vi "rszvl_core_global.vi"() -> ()   [LabVIEW 2014] (continued)
"*WAI"=FALSE}, "Check Status Callback"=""}, {"Level"=3, "Descriptive Name"="NWA Distance To Fault Auto Number Of Points", "Class Only"=FALSE, "Data Type"=4, "Access"=1, "Identifier"="RSZVL_ATTR_NWA_DFAULT_POINTS", "Range Table"="", "Command"="CALC{Channel}:TRAN:DTF:POIN", "Read Callback"="", "Write Callback"="", "Range Callback"="", "Check Callback"="", "Rngtable Callback"="", "Coerce Callback"="", "User Callback"="", "Supported Models"="", "Instrument Options"="", "Repeated Capabilities"="", "Restricted Repeated Capabilities"="", "Help"="This attribute starts the automatic calculation of the number of points.\n\nAvailable Repeated Capabilities:\nChannel: CH1,CH2,CH3,CH4,CH5,CH6,CH7,CH8,CH9,CH10,CH11,CH12,CH13,CH14,CH15,CH16,CH17,CH18,CH19,CH20\r\n\nRemote-control command(s):\nCALCulate<Chn>:TRANsform:DTFault:POINts", "Flags"={"OPC Wait"=FALSE, "Dont check status"=FALSE, "*WAI"=FALSE}, "Check Status Callback"=""}, {"Level"=3, "Descriptive Name"="NWA Distance To Fault Select Cable", "Class Only"=FALSE, "Data Type"=2, "Access"=2, "Identifier"="RSZVL_ATTR_NWA_DFAULT_SELECT_CABLE", "Range Table"="", "Command"="CALC{Channel}:TRAN:DTF:SEL", "Read Callback"="", "Write Callback"="rszvl_quotedString_WriteCallback.vi", "Range Callback"="", "Check Callback"="", "Rngtable Callback"="", "Coerce Callback"="", "User Callback"="", "Supported Models"="", "Instrument Options"="", "Repeated Capabilities"="", "Restricted Repeated Capabilities"="", "Help"="This attribute selects a standard cable or a previously defined cable identified by its name.\n\nAvailable Repeated Capabilities:\nChannel: CH1,CH2,CH3,CH4,CH5,CH6,CH7,CH8,CH9,CH10,CH11,CH12,CH13,CH14,CH15,CH16,CH17,CH18,CH19,CH20\r\n\nRemote-control command(s):\nCALCulate<Chn>:TRANsform:DTFault:SELect '<cable name>'", "Flags"={"OPC Wait"=FALSE, "Dont check status"=FALSE, "*WAI"=FALSE}, "Check Status Callback"=""}, {"Level"=3, "Descriptive Name"="NWA Distance To Fault Delete Cable", "Class Only"=FALSE, "Data Type"=2, "Access"=1, "Identifier"="RSZVL_ATTR_NWA_DFAULT_DELETE_CABLE", "Range Table"="", "Command"="CALC{Channel}:TRAN:DTF:DEL", "Read Callback"="rszvl_quotedString_ReadCallback.vi", "Write Callback"="rszvl_quotedString_WriteCallback.vi", "Range Callback"="", "Check Callback"="", "Rngtable Callback"="", "Coerce Callback"="", "User Callback"="", "Supported Models"="", "Instrument Options"="", "Repeated Capabilities"="", "Restricted Repeated Capabilities"="", "Help"="This attribute deletes a previously defined cable identified by its name.\n\nAvailable Repeated Capabilities:\nChannel: CH1,CH2,CH3,CH4,CH5,CH6,CH7,CH8,CH9,CH10,CH11,CH12,CH13,CH14,CH15,CH16,CH17,CH18,CH19,CH20\r\n\nRemote-control command(s):\nCALCulate<Chn>:TRANsform:DTFault:DELete '<cable name>'", "Flags"={"OPC Wait"=FALSE, "Dont check status"=FALSE, "*WAI"=FALSE}, "Check Status Callback"=""}, {"Level"=3, "Descriptive Name"="NWA Distance To Fault Save Cable", "Class Only"=FALSE, "Data Type"=2, "Access"=1, "Identifier"="RSZVL_ATTR_NWA_DFAULT_SAVE_CABLE", "Range Table"="", "Command"="MMEM:STOR:CABL", "Read Callback"="", "Write Callback"="rszvl_quotedString_WriteCallback.vi", "Range Callback"="", "Check Callback"="", "Rngtable Callback"="", "Coerce Callback"="", "User Callback"="", "Supported Models"="", "Instrument Options"="", "Repeated Capabilities"="", "Restricted Repeated Capabilities"="", "Help"="This attribute copies all pre-defined and user-defined cable description files (*.rsc) to a specified directory. The contents of the source directories for cable description files (C:\\R_S\\Instr\\resources\\Nwa\\CableTypes for predefined, C:\\R_S\\Instr\\user\\Nwa\\CableTypes for user-defined cables) are not affected.\n\nAvailable Repeated Capabilities:\nNone\n\nRemote-control command(s):\nMMEMory:STORe:CABLe '<target_directory>'", "Flags"={"OPC Wait"=FALSE, "Dont check status"=FALSE, "*WAI"=FALSE}, "Check Status Callback"=""}, {"Level"=3, "Descriptive Name"="NWA Distance To Fault Load Cable", "Class Only"=FALSE, "Data Type"=2, "Access"=1, "Identifier"="RSZVL_ATTR_NWA_DFAULT_LOAD_CABLE", "Range Table"="", "Command"="MMEM:LOAD:CABL", "Read Callback"="", "Write Callback"="rszvl_quotedString_WriteCallback.vi", "Range Callback"="", "Check Callback"="", "Rngtable Callback"="", "Coerce Callback"="", "User Callback"="", "Supported Models"="", "Instrument Options"="", "Repeated Capabilities"="", "Restricted Repeated Capabilities"="", "Help"="This attribute loads all cable description files (*.rsc) from a specified directory. The default source directories for cable\ndescription files (C:\\R_S\\Instr\\resources\\Nwa\\CableTypes for predefined, C:\\R_S\\Instr\\user\\Nwa\\CableTypes for user-defined cables) are not affected.\n\nAvailable Repeated Capabilities:\nNone\n\nRemote-control command(s):\nMMEMory:LOAD:CABLe '<source_directory>'", "Flags"={"OPC Wait"=FALSE, "Dont check status"=FALSE, "*WAI"=FALSE}, "Check Status Callback"=""}, {"Level"=3, "Descriptive Name"="Fault Limit Check", "Class Only"=TRUE, "Data Type"=0, "Access"=0, "Identifier"="", "Range Table"="", "Command"="", "Read Callback"="", "Write Callback"="", "Range Callback"="", "Check Callback"="", "Rngtable Callback"="", "Coerce Callback"="", "User Callback"="", "Supported Models"="", "Instrument Options"="", "Repeated Capabilities"="", "Restricted Repeated Capabilities"="", "Help"="Put a help here", "Flags"={"OPC Wait"=FALSE, "Dont check status"=FALSE, "*WAI"=FALSE}, "Check Status Callback"=""}, {"Level"=4, "Descriptive Name"="NWA Fault Limit Check", "Class Only"=FALSE, "Data Type"=3, "Access"=2, "Identifier"="RSZVL_ATTR_NWA_FAULT_LIMIT_CHECK", "Range Table"="", "Command"="CALC{Channel}:TRAN:DTF:PEAK:STAT", "Read Callback"="", "Write Callback"="", "Range Callback"="", "Check Callback"="", "Rngtable Callback"="", "Coerce Callback"="", "User Callback"="", "Supported Models"="", "Instrument Options"="", "Repeated Capabilities"="", "Restricted Repeated Capabilities"="", "Help"="This attribute enables or disables the fault limit check.\n\nAvailable Repeated Capabilities:\nChannel: CH1,CH2,CH3,CH4,CH5,CH6,CH7,CH8,CH9,CH10,CH11,CH12,CH13,CH14,CH15,CH16,CH17,CH18,CH19,CH20\r\n\nRemote-control command(s):\nCALCulate<Chn>:TRANsform:DTFault:PEAK:STATe ON | OFF", "Flags"={"OPC Wait"=FALSE, "Dont check status"=FALSE, "*WAI"=FALSE}, "Check Status Callback"=""}, {"Level"=4, "Descriptive Name"="NWA Fault Threshold", "Class Only"=FALSE, "Data Type"=1, "Access"=2, "Identifier"="RSZVL_ATTR_NWA_FAULT_THRESHOLD", "Range Table"="", "Command"="CALC{Channel}:TRAN:DTF:PEAK:THR", "Read Callback"="", "Write Callback"="", "Range Callback"="", "Check Callback"="", "Rngtable Callback"="", "Coerce Callback"="", "User Callback"="", "Supported Models"="", "Instrument Options"="", "Repeated Capabilities"="", "Restricted Repeated Capabilities"="", "Help"="This attribute specify a fault limit.\n\nAvailable Repeated Capabilities:\nChannel: CH1,CH2,CH3,CH4,CH5,CH6,CH7,CH8,CH9,CH10,CH11,CH12,CH13,CH14,CH15,CH16,CH17,CH18,CH19,CH20\r\n\nRemote-control command(s):\nCALCulate<Chn>:TRANsform:DTFault:PEAK:THReshold", "Flags"={"OPC Wait"=FALSE, "Dont check status"=FALSE, "*WAI"=FALSE}, "Check Status Callback"=""}, {"Level"=4, "Descriptive Name"="NWA Fault Peak Count", "Class Only"=FALSE, "Data Type"=0, "Access"=0, "Identifier"="RSZVL_ATTR_NWA_FAULT_PEAK_COUNT", "Range Table"="", "Command"="CALC{Channel}:TRAN:DTF:PEAK:COUN?", "Read Callback"="", "Write Callback"="", "Range Callback"="", "Check Callback"="", "Rngtable Callback"="", "Coerce Callback"="", "User Callback"="", "Supported Models"="", "Instrument Options"="", "Repeated Capabilities"="", "Restricted Repeated Capabilities"="", "Help"="This attribute returns the number of peaks on the active distance trace which are above the fault limit (CALCulate<Chn>:TRANsform:DTFault:PEAK:THReshold).\n\nAvailable Repeated Capabilities:\nChannel: CH1,CH2,CH3,CH4,CH5,CH6,CH7,CH8,CH9,CH10,CH11,CH12,CH13,CH14,CH15,CH16,CH17,CH18,CH19,CH20\r\n\nRemote-control command(s):\nCALCulate<Chn>:TRANsform:DTFault:PEAK:COUNt?", "Flags"={"OPC Wait"=FALSE, "Dont check status"=FALSE, "*WAI"=FALSE}, "Check Status Callback"=""}, {"Level"=1, "Descriptive Name"="NWA Display Control", "Class Only"=TRUE, "Data Type"=0, "Access"=0, "Identifier"="", "Range Table"="", "Command"="", "Read Callback"="", "Write Callback"="", "Range Callback"="", "Check Callback"="", "Rngtable Callback"="", "Coerce Callback"="", "User Callback"="", "Supported Models"="", "Instrument Options"="", "Repeated Capabilities"="", "Restricted Repeated Capabilities"="", "Help"="(1) NWA Color Scheme:\nThis attribute selects the color scheme for all diagram areas in the active setup.\n\n(2) NWA Frequency Info State:\nThis attribute activates/deactivates the display of the frequency information. For example to protect confidential data it can be useful to hide the frequency information.\n\n(3) NWA Trace Color State:\nThis attribute defines the trace color schemes in different diagram areas.\n\n(4) NWA Marker Color State:\nThis attribute displays all markers with the same color or display each marker with the color of the associated trace.\n\n(5) NWA Save Color Scheme:\nThis attribute stores a color scheme to a specified NWA color scheme file.\n\n(6) NWA Load Color Scheme:\nThis attribute loads a color scheme from a specified NWA color scheme file.\n\n(7) NWA Display Update:\nThis attribute switches the display on or off while the analyzer is in the remote state. The attribute has no effect while the analyzer is in the Local operating state.\n\n(8) NWA Error Display State:\nThis attribute switches the display of a tooltip for remote command errors on or off. The tooltip appears at the bottom of the remote screen and of the manual screen.\n\n(9) NWA Remote Display Title:\nThis attribute defines a title for the remote display.\n\n(10) NWA Diagram Area State:\nThis attribute creates or deletes a diagram area, identified by its area number <Wnd>.\n\n(11) NWA Diagram Area Maximize:\nThis attribute maximizes all diagram areas in the active setup or restores the previous display configuration. It acts on all diagrams of the current setup, however, the diagram no. <Wnd> is displayed on top of the others.\n\n(12) NWA Diagram Area Title State:\nThis attribute displays or hides the title for area number <Wnd>, defined by means of DISPlay:WINDow<Wnd>:TITLe:DATA.\n\n(13) NWA Diagram Area Title:\nThis attribute defines a title for diagram area <Wnd>.", "Flags"={"OPC Wait"=FALSE, "Dont check status"=FALSE, "*WAI"=FALSE}, "Check Status Callback"=""}, {"Level"=2, "Descriptive Name"="NWA Color Scheme", "Class Only"=FALSE, "Data Type"=0, "Access"=2, "Identifier"="RSZVL_ATTR_NWA_COLOR_SCHEME", "Range Table"="rszvl_rngNWAColorScheme", "Command"="SYST:DISP:COL", "Read Callback"="", "Write Callback"="", "Range Callback"="", "Check Callback"="", "Rngtable Callback"="", "Coerce Callback"="", "User Callback"="", "Supported Models"="", "Instrument Options"="", "Repeated Capabilities"="", "Restricted Repeated Capabilities"="", "Help"="This attribute selects the color scheme for all diagram areas in the active setup.\n\nAvailable Repeated Capabilities:\nNone\n\nRemote-control command(s):\nSYSTem:DISPlay:COLor DBACkground | LBACkground | BWLStyles | BWSolid", "Flags"={"OPC Wait"=FALSE, "Dont check status"=FALSE, "*WAI"=FALSE}, "Check Status Callback"=""}, {"Level"=2, "Descriptive Name"="NWA Frequency Info State", "Class Only"=FALSE, "Data Type"=3, "Access"=2, "Identifier"="RSZVL_ATTR_NWA_FREQ_INFO_STATE", "Range Table"="", "Command"="DISP:ANN:FREQ:STAT", "Read Callback"="", "Write Callback"="", "Range Callback"="", "Check Callback"="", "Rngtable Callback"="", "Coerce Callback"="", "User Callback"="", "Supported Models"="", "Instrument Options"="", "Repeated Capabilities"="", "Restricted Repeated Capabilities"="", "Help"="This attribute activates/deactivates the display of the frequency information. For example to protect confidential data it can be useful to hide the frequency information.\n\nAvailable Repeated Capabilities:\nNone\n\nRemote-control command(s):\nDISPlay:ANNotation:FREQuency[:STATe] ON | OFF", "Flags"={"OPC Wait"=FALSE, "Dont check status"=FALSE, "*WAI"=FALSE}, "Check Status Callback"=""}, {"Level"=2, "Descriptive Name"="NWA Trace Color State", "Class Only"=FALSE, "Data Type"=3, "Access"=2, "Identifier"="RSZVL_ATTR_NWA_TRACE_COLOR_STATE", "Range Table"="", "Command"="DISP:CMAP:TRAC:COL:STAT", "Read Callback"="", "Write Callback"="", "Range Callback"="", "Check Callback"="", "Rngtable Callback"="", "Coerce Callback"="", "User Callback"="", "Supported Models"="", "Instrument Options"="", "Repeated Capabilities"="", "Restricted Repeated Capabilities"="", "Help"="This attribute defines the trace color schemes in different diagram areas.\n\nAvailable Repeated Capabilities:\nNone\n\nRemote-control command(s):\nDISPlay:CMAP<Element>:TRACe:COLor[:STATe] ON | OFF", "Flags"={"OPC Wait"=FALSE, "Dont check status"=FALSE, "*WAI"=FALSE}, "Check Status Callback"=""}, {"Level"=2, "Descriptive Name"="NWA Marker Color State", "Class Only"=FALSE, "Data Type"=3, "Access"=2, "Identifier"="RSZVL_ATTR_NWA_MARKER_COLOR_STATE", "Range Table"="", "Command"="DISP:CMAP:MARK:STAT", "Read Callback"="", "Write Callback"="", "Range Callback"="", "Check Callback"="", "Rngtable Callback"="", "Coerce Callback"="", "User Callback"="", "Supported Models"="", "Instrument Options"="", "Repeated Capabilities"="", "Restricted Repeated Capabilities"="", "Help"="This attribute displays all markers with the same color or display each marker with the color of the associated trace.\n\nAvailable Repeated Capabilities:\nNone\n\nRemote-control command(s):\nDISPlay:CMAP<Element>:MARKer[:STATe] ON | OFF", "Flags"={"OPC Wait"=FALSE, "Dont check status"=FALSE, "*WAI"=FALSE}, "Check Status Callback"=""}, {"Level"=2, "Descriptive Name"="NWA Save Color Scheme", "Class Only"=FALSE, "Data Type"=2, "Access"=1, "Identifier"="RSZVL_ATTR_NWA_SAVE_COLOR_SCHEME", "Range Table"="", "Command"="MMEM:STOR:CMAP", "Read Callback"="", "Write Callback"="rszvl_quotedString_WriteCallback.vi", "Range Callback"="", "Check Callback"="", "Rngtable Callback"="", "Coerce Callback"="", "User Callback"="", "Supported Models"="", "Instrument Options"="", "Repeated Capabilities"="", "Restricted Repeated Capabilities"="", "Help"="This attribute stores a color scheme to a specified NWA color scheme file.\n\nAvailable Repeated Capabilities:\nNone\n\nRemote-control command(s):\nMMEMory:STORe:CMAP '<file_name>'", "Flags"={"OPC Wait"=FALSE, "Dont check status"=FALSE, "*WAI"=FALSE}, "Check Status Callback"=""}, {"Level"=2, "Descriptive Name"="NWA Load Color Scheme", "Class Only"=FALSE, "Data Type"=2, "Access"=1, "Identifier"="RSZVL_ATTR_NWA_LOAD_COLOR_SCHEME", "Range Table"="", "Command"="MMEM:LOAD:CMAP", "Read Callback"="", "Write Callback"="rszvl_quotedString_WriteCallback.vi", "Range Callback"="", "Check Callback"="", "Rngtable Callback"="", "Coerce Callback"="", "User Callback"="", "Supported Models"="", "Instrument Options"="", "Repeated Capabilities"="", "Restricted Repeated Capabilities"="", "Help"="This attribute loads a color scheme from a specified NWA color scheme file.\n\nAvailable Repeated Capabilities:\nNone\n\nRemote-control command(s):\nMMEMory:LOAD:CMAP '<file_name>'", "Flags"={"OPC Wait"=FALSE, "Dont check status"=FALSE, "*WAI"=FALSE}, "Check Status Callback"=""}, {"Level"=2, "Descriptive Name"="NWA Display Update", "Class Only"=FALSE, "Data Type"=3, "Access"=2, "Identifier"="RSZVL_ATTR_NWA_DISPLAY_UPDATE", "Range Table"="", "Command"="SYST:DISP:UPD", "Read Callback"="", "Write Callback"="", "Range Callback"="", "Check Callback"="", "Rngtable Callback"="", "Coerce Callback"="", "User Callback"="", "Supported Models"="", "Instrument Options"="", "Repeated Capabilities"="", "Restricted Repeated Capabilities"="", "Help"="This attribute switches the display on or off while the analyzer is in the remote state. The attribute has no effect while the analyzer is in the Local operating state.\n\nAvailable Repeated Capabilities:\nNone\n\nRemote-control command(s):\nSYSTem:DISPlay:UPDate ON | OFF", "Flags"={"OPC Wait"=FALSE, "Dont check status"=FALSE, "*WAI"=FALSE}, "Check Status Callback"=""}, {"Level"=2, "Descriptive Name"="NWA Error Display State", "Class Only"=FALSE, "Data Type"=3, "Access"=2, "Identifier"="RSZVL_ATTR_NWA_ERROR_DISPLAY_STATE", "Range Table"="", "Command"="SYST:ERR:DISP", "Read Callback"="", "Write Callback"="", "Range Callback"="", "Check Callback"="", "Rngtable Callback"="", "Coerce Callback"="", "User Callback"="", "Supported Models"="", "Instrument Options"="", "Repeated Capabilities"="", "Restricted Repeated Capabilities"="", "Help"="This attribute switches the display of a tooltip for remote command errors on or off. The tooltip appears at the bottom of the remote screen and of the manual screen.\n\nAvailable Repeated Capabilities:\nNone\n\nRemote-control command(s):\nSYSTem:ERRor:DISPlay ON | OFF", "Flags"={"OPC Wait"=FALSE, "Dont check status"=FALSE, "*WAI"=FALSE}, "Check Status Callback"=""}, {"Level"=2, "Descriptive Name"="NWA Remote Display Title", "Class Only"=FALSE, "Data Type"=2, "Access"=2, "Identifier"="RSZVL_ATTR_NWA_REMOTE_DISPLAY_TITLE", "Range Table"="", "Command"="SYST:USER:DISP:TITL", "Read Callback"="rszvl_quotedString_ReadCallback.vi", "Write Callback"="rszvl_quotedString_WriteCallback.vi", "Range Callback"="", "Check Callback"="", "Rngtable Callback"="", "Coerce Callback"="", "User Callback"="", "Supported Models"="", "Instrument Options"="", "Repeated Capabilities"="", "Restricted Repeated Capabilities"="", "Help"="This attribute defines a title for the remote display.\n\nAvailable Repeated Capabilities:\nNone\n\nRemote-control command(s):\nSYSTem:USER:DISPlay:TITLe '<title>'", "Flags"={"OPC Wait"=FALSE, "Dont check status"=FALSE, "*WAI"=FALSE}, "Check Status Callback"=""}, {"Level"=2, "Descriptive Name"="NWA Diagram Area State", "Class Only"=FALSE, "Data Type"=3, "Access"=2, "Identifier"="RSZVL_ATTR_NWA_DIAGRAM_AREA_STATE", "Range Table"="", "Command"="DISP:WIND{DiagramArea}:STAT", "Read Callback"="", "Write Callback"="", "Range Callback"="", "Check Callback"="", "Rngtable Callback"="", "Coerce Callback"="", "User Callback"="", "Supported Models"="", "Instrument Options"="", "Repeated Capabilities"="", "Restricted Repeated Capabilities"="", "Help"="This attribute creates or deletes a diagram area, identified by its area number <Wnd>.\n\nAvailable Repeated Capabilities:\nDiagramArea: DA1,DA2,DA3,DA4,DA5,DA6,DA7,DA8,DA9,DA10\r\n\nRemote-control command(s):\nDISPlay[:WINDow<Wnd>]:STATe ON | OFF", "Flags"={"OPC Wait"=FALSE, "Dont check status"=FALSE, "*WAI"=FALSE}, "Check Status Callback"=""}, {"Level"=2, "Descriptive Name"="NWA Diagram Area Maximize", "Class Only"=FALSE, "Data Type"=3, "Access"=2, "Identifier"="RSZVL_ATTR_NWA_DIAGRAM_AREA_MAXIMIZE", "Range Table"="", "Command"="DISP:WIND{DiagramArea}:MAX", "Read Callback"="", "Write Callback"="", "Range Callback"="", "Check Callback"="", "Rngtable Callback"="", "Coerce Callback"="", "User Callback"="", "Supported Models"="", "Instrument Options"="", "Repeated Capabilities"="", "Restricted Repeated Capabilities"="", "Help"="This attribute maximizes all diagram areas in the active setup or restores the previous display configuration. It acts on all diagrams of the current setup, however, the diagram no. <Wnd> is displayed on top of the others.\n\nAvailable Repeated Capabilities:\nDiagramArea: DA1,DA2,DA3,DA4,DA5,DA6,DA7,DA8,DA9,DA10\r\n\nRemote-control command(s):\nDISPlay[:WINDow<Wnd>]:MAXimize ON | OFF", "Flags"={"OPC Wait"=FALSE, "Dont check status"=FALSE, "*WAI"=FALSE}, "Check Status Callback"=""}, {"Level"=2, "Descriptive Name"="NWA Diagram Area Title State", "Class Only"=FALSE, "Data Type"=3, "Access"=2, "Identifier"="RSZVL_ATTR_NWA_DIAGRAM_AREA_TITLE_STATE", "Range Table"="", "Command"="DISP:WIND{DiagramArea}:TITL:STAT", "Read Callback"="", "Write Callback"="", "Range Callback"="", "Check Callback"="", "Rngtable Callback"="", "Coerce Callback"="", "User Callback"="", "Supported Models"="", "Instrument Options"="", "Repeated Capabilities"="", "Restricted Repeated Capabilities"="", "Help"="This attribute displays or hides the title for area number <Wnd>, defined by means of DISPlay:WINDow<Wnd>:TITLe:DATA.\n\nAvailable Repeated Capabilities:\nDiagramArea: DA1,DA2,DA3,DA4,DA5,DA6,DA7,DA8,DA9,DA10\r\n\nRemote-control command(s):\nDISPlay[:WINDow<Wnd>]:TITLe[:STATe] ON | OFF", "Flags"={"OPC Wait"=FALSE, "Dont check status"=FALSE, "*WAI"=FALSE}, "Check Status Callback"=""}, {"Level"=2, "Descriptive Name"="NWA Diagram Area Title", "Class Only"=FALSE, "Data Type"=2, "Access"=2, "Identifier"="RSZVL_ATTR_NWA_DIAGRAM_AREA_TITLE", "Range Table"="", "Command"="DISP:WIND{DiagramArea}:TITL:DATA", "Read Callback"="rszvl_quotedString_ReadCallback.vi", "Write Callback"="rszvl_quotedString_WriteCallback.vi", "Range Callback"="", "Check Callback"="", "Rngtable Callback"="", "Coerce Callback"="", "User Callback"="", "Supported Models"="", "Instrument Options"="", "Repeated Capabilities"="", "Restricted Repeated Capabilities"="", "Help"="This attribute defines a title for diagram area <Wnd>.\n\nAvailable Repeated Capabilities:\nDiagramArea: DA1,DA2,DA3,DA4,DA5,DA6,DA7,DA8,DA9,DA10\r\n\nRemote-control command(s):\nDISPlay[:WINDow<Wnd>]:TITLe:DATA '<string>'", "Flags"={"OPC Wait"=FALSE, "Dont check status"=FALSE, "*WAI"=FALSE}, "Check Status Callback"=""}, {"Level"=1, "Descriptive Name"="NWA Setup Select", "Class Only"=TRUE, "Data Type"=0, "Access"=0, "Identifier"="", "Range Table"="", "Command"="", "Read Callback"="", "Write Callback"="", "Range Callback"="", "Check Callback"="", "Rngtable Callback"="", "Coerce Callback"="", "User Callback"="", "Supported Models"="", "Instrument Options"="", "Repeated Capabilities"="", "Restricted Repeated Capabilities"="", "Help"="(1) NWA Create New Setup:\nThis attribute creates a new setup <setup_name> using default settings for the traces, channels and diagram areas. The created setup becomes the active setup.\n\n(2) NWA Select Setup:\nThis attribute selects a setup as the active setup.\n\n(3) NWA Close Setup:\nThis attribute closes the specified setup.", "Flags"={"OPC Wait"=FALSE, "Dont check status"=FALSE, "*WAI"=FALSE}, "Check Status Callback"=""}, {"Level"=2, "Descriptive Name"="NWA Create New Setup", "Class Only"=FALSE, "Data Type"=2, "Access"=1, "Identifier"="RSZVL_ATTR_NWA_CREATE_NEW_SETUP", "Range Table"="", "Command"="MEM:DEF", "Read Callback"="", "Write Callback"="rszvl_quotedString_WriteCallback.vi", "Range Callback"="", "Check Callback"="", "Rngtable Callback"="", "Coerce Callback"="", "User Callback"="", "Supported Models"="", "Instrument Options"="", "Repeated Capabilities"="", "Restricted Repeated Capabilities"="", "Help"="This attribute creates a new setup <setup_name> using default settings for the traces, channels and diagram areas. The created setup becomes the active setup.\n\nAvailable Repeated Capabilities:\nNone\n\nRemote-control command(s):\nMEMory:DEFine '<setup_name>'", "Flags"={"OPC Wait"=FALSE, "Dont check status"=FALSE, "*WAI"=FALSE}, "Check Status Callback"=""}, {"Level"=2, "Descriptive Name"="NWA Select Setup", "Class Only"=FALSE, "Data Type"=2, "Access"=1, "Identifier"="RSZVL_ATTR_NWA_SELECT_SETUP", "Range Table"="", "Command"="MEM:SEL", "Read Callback"="", "Write Callback"="rszvl_quotedString_WriteCallback.vi", "Range Callback"="", "Check Callback"="", "Rngtable Callback"="", "Coerce Callback"="", "User Callback"="", "Supported Models"="", "Instrument Options"="", "Repeated Capabilities"="", "Restricted Repeated Capabilities"="", "Help"="This attribute selects a setup as the active setup.\n\nAvailable Repeated Capabilities:\nNone\n\nRemote-control command(s):\nMEMory:SELect '<setup_name>'", "Flags"={"OPC Wait"=FALSE, "Dont check status"=FALSE, "*WAI"=FALSE}, "Check Status Callback"=""}, {"Level"=2, "Descriptive Name"="NWA Close Setup", "Class Only"=FALSE, "Data Type"=2, "Access"=1, "Identifier"="RSZVL_ATTR_NWA_CLOSE_SETUP", "Range Table"="", "Command"="MEM:DEL:NAME", "Read Callback"="", "Write Callback"="rszvl_quotedString_WriteCallback.vi", "Range Callback"="", "Check Callback"="", "Rngtable Callback"="", "Coerce Callback"="", "User Callback"="", "Supported Models"="", "Instrument Options"="", "Repeated Capabilities"="", "Restricted Repeated Capabilities"="", "Help"="This attribute closes the specified setup.\n\nAvailable Repeated Capabilities:\nNone\n\nRemote-control command(s):\nMEMory:DELete[:NAME] '<file_name>'", "Flags"={"OPC Wait"=FALSE, "Dont check status"=FALSE, "*WAI"=FALSE}, "Check Status Callback"=""}, {"Level"=1, "Descriptive Name"="NWA File", "Class Only"=TRUE, "Data Type"=0, "Access"=0, "Identifier"="", "Range Table"="", "Command"="", "Read Callback"="", "Write Callback"="", "Range Callback"="", "Check Callback"="", "Rngtable Callback"="", "Coerce Callback"="", "User Callback"="", "Supported Models"="", "Instrument Options"="", "Repeated Capabilities"="", "Restricted Repeated Capabilities"="", "Help"="(1) NWA Load Setup:\nThis attribute loads configuration data from a specified setup file and sets the analyzer to the corresponding instrument state.\n\n(2) NWA Save Setup:\nThis attribute stores the configuration data of the current setup to a specified setup file.", "Flags"={"OPC Wait"=FALSE, "Dont check status"=FALSE, "*WAI"=FALSE}, "Check Status Callback"=""}, {"Level"=2, "Descriptive Name"="NWA Load Setup", "Class Only"=FALSE, "Data Type"=2, "Access"=1, "Identifier"="RSZVL_ATTR_NWA_LOAD_SETUP", "Range Table"="", "Command"="MMEM:LOAD:NWAN", "Read Callback"="", "Write Callback"="rszvl_FileStateSpecialFormat_WriteCallback.vi", "Range Callback"="", "Check Callback"="", "Rngtable Callback"="", "Coerce Callback"="", "User Callback"="", "Supported Models"="", "Instrument Options"="", "Repeated Capabilities"="", "Restricted Repeated Capabilities"="", "Help"="This attribute loads configuration data from a specified setup file and sets the analyzer to the corresponding instrument state.\n\nAvailable Repeated Capabilities:\nNone\n\nRemote-control command(s):\nMMEMory:LOAD:NWANalyzer 1,'<file_name>'", "Flags"={"OPC Wait"=FALSE, "Dont check status"=FALSE, "*WAI"=FALSE}, "Check Status Callback"=""}, {"Level"=2, "Descriptive Name"="NWA Save Setup", "Class Only"=FALSE, "Data Type"=2, "Access"=1, "Identifier"="RSZVL_ATTR_NWA_SAVE_SETUP", "Range Table"="", "Command"="MMEM:STOR:NWAN", "Read Callback"="", "Write Callback"="rszvl_FileStateSpecialFormat_WriteCallback.vi", "Range Callback"="", "Check Callback"="", "Rngtable Callback"="", "Coerce Callback"="", "User Callback"="", "Supported Models"="", "Instrument Options"="", "Repeated Capabilities"="", "Restricted Repeated Capabilities"="", "Help"="This attribute stores the configuration data of the current setup to a specified setup file.\n\nAvailable Repeated Capabilities:\nNone\n\nRemote-control command(s):\nMMEMory:STORe:NWANalyzer 1,'<file_name>'", "Flags"={"OPC Wait"=FALSE, "Dont check status"=FALSE, "*WAI"=FALSE}, "Check Status Callback"=""}, {"Level"=1, "Descriptive Name"="NWA System", "Class Only"=TRUE, "Data Type"=0, "Access"=0, "Identifier"="", "Range Table"="", "Command"="", "Read Callback"="", "Write Callback"="", "Range Callback"="", "Check Callback"="", "Rngtable Callback"="", "Coerce Callback"="", "User Callback"="", "Supported Models"="", "Instrument Options"="", "Repeated Capabilities"="", "Restricted Repeated Capabilities"="", "Help"="(1) NWA System Preset Scope:\nThis attribute specifies whether a preset (SYSTem:PRESet; *RST) affects the active setup only or all open setups. This attribute is effective in the Network Analyzer mode only and returns an error in other modes.\n\n\n(2) NWA User Preset State:\nThis attribute selects a factory preset or a user-defined preset.\n\n(3) NWA User Preset Name:\nThis attribute specifies the name of a setup file (.nwa) to be used for a user-defined preset.\n\n(4) NWA System Settings Update:\nThis attribute initiates an immediate update of the channel or trace settings. The atttribute has an effect if the analyzer operates in single sweep mode (INITiate<Ch>:CONTinuous OFF) and if the display update is switched off (SYSTem:DISPlay:UPDate OFF). \n\n(5) NWA System Lock Keys:\nThis attribute locks or unlocks the local controls of the analyzer. This includes the front panel keys, the keyboard, or other local interfaces.\n\n(6) NWA Alarm Sound State:\nThis attribute switches alarm sounds on or off. \n\n(7) NWA Status Sound State:\nThis attribute switches status sounds on or off.", "Flags"={"OPC Wait"=FALSE, "Dont check status"=FALSE, "*WAI"=FALSE}, "Check Status Callback"=""}, {"Level"=2, "Descriptive Name"="NWA System Preset Scope", "Class Only"=FALSE, "Data Type"=0, "Access"=2, "Identifier"="RSZVL_ATTR_NWA_SYSTEM_PRESET_SCOPE", "Range Table"="rszvl_rngNWAPresetScope", "Command"="SYST:PRES:SCOP", "Read Callback"="", "Write Callback"="", "Range Callback"="", "Check Callback"="", "Rngtable Callback"="", "Coerce Callback"="", "User Callback"="", "Supported Models"="", "Instrument Options"="", "Repeated Capabilities"="", "Restricted Repeated Capabilities"="", "Help"="This attribute specifies whether a preset (SYSTem:PRESet; *RST) affects the active setup only or all open setups. This attribute is effective in the Network Analyzer mode only and returns an error in other modes.\n\nAvailable Repeated Capabilities:\nNone\n\nRemote-control command(s):\nSYSTem:PRESet:SCOPe ALL | SINGle", "Flags"={"OPC Wait"=FALSE, "Dont check status"=FALSE, "*WAI"=FALSE}, "Check Status Callback"=""}, {"Level"=2, "Descriptive Name"="NWA User Preset State", "Class Only"=FALSE, "Data Type"=3, "Access"=2, "Identifier"="RSZVL_ATTR_NWA_USER_PRESET_STATE", "Range Table"="", "Command"="SYST:PRES:USER:STAT", "Read Callback"="", "Write Callback"="", "Range Callback"="", "Check Callback"="", "Rngtable Callback"="", "Coerce Callback"="", "User Callback"="", "Supported Models"="", "Instrument Options"="", "Repeated Capabilities"="", "Restricted Repeated Capabilities"="", "Help"="This attribute selects a factory preset or a user-defined preset.\n\nAvailable Repeated Capabilities:\nNone\n\nRemote-control command(s):\nSYSTem:PRESet:USER[:STATe] ON | OFF", "Flags"={"OPC Wait"=FALSE, "Dont check status"=FALSE, "*WAI"=FALSE}, "Check Status Callback"=""}, {"Level"=2, "Descriptive Name"="NWA User Preset Name", "Class Only"=FALSE, "Data Type"=2, "Access"=2, "Identifier"="RSZVL_ATTR_NWA_USER_PRESET_NAME", "Range Table"="", "Command"="SYST:PRES:USER:NAME", "Read Callback"="rszvl_quotedString_ReadCallback.vi", "Write Callback"="rszvl_quotedString_WriteCallback.vi", "Range Callback"="", "Check Callback"="", "Rngtable Callback"="", "Coerce Callback"="", "User Callback"="", "Supported Models"="", "Instrument Options"="", "Repeated Capabilities"="", "Restricted Repeated Capabilities"="", "Help"="This attribute specifies the name of a setup file (.nwa) to be used for a user-defined preset.\n\nAvailable Repeated Capabilities:\nNone\n\nRemote-control command(s):\nSYSTem:PRESet:USER:NAME '<Setup_file>'", "Flags"={"OPC Wait"=FALSE, "Dont check status"=FALSE, "*WAI"=FALSE}, "Check Status Callback"=""}, {"Level"=2, "Descriptive Name"="NWA System Settings Update", "Class Only"=FALSE, "Data Type"=4, "Access"=1, "Identifier"="RSZVL_ATTR_NWA_SYSTEM_SETTINGS_UPDATE", "Range Table"="", "Command"="SYST:SETT:UPD ONCE", "Read Callback"="", "Write Callback"="", "Range Callback"="", "Check Callback"="", "Rngtable Callback"="", "Coerce Callback"="", "User Callback"="", "Supported Models"="", "Instrument Options"="", "Repeated Capabilities"="", "Restricted Repeated Capabilities"="", "Help"="This attribute initiates an immediate update of the channel or trace settings. The atttribute has an effect if the analyzer operates in single sweep mode (INITiate<Ch>:CONTinuous OFF) and if the display update is switched off (SYSTem:DISPlay:UPDate OFF).\n\nAvailable Repeated Capabilities:\nNone\n\nRemote-control command(s):\nSYSTem:SETTings:UPDate ONCE", "Flags"={"OPC Wait"=FALSE, "Dont check status"=FALSE, "*WAI"=FALSE}, "Check Status Callback"=""}, {"Level"=2, "Descriptive Name"="NWA System Lock Keys", "Class Only"=FALSE, "Data Type"=3, "Access"=2, "Identifier"="RSZVL_ATTR_NWA_SYSTEM_KLOCK", "Range Table"="", "Command"="SYST:KLOC", "Read Callback"="", "Write Callback"="", "Range Callback"="", "Check Callback"="", "Rngtable Callback"="", "Coerce Callback"="", "User Callback"="", "Supported Models"="", "Instrument Options"="", "Repeated Capabilities"="", "Restricted Repeated Capabilities"="", "Help"="This attribute locks or unlocks the local controls of the analyzer. This includes the front panel keys, the keyboard, or other local interfaces.\n\nAvailable Repeated Capabilities:\nNone\n\nRemote-control command(s):\nSYSTem:KLOCk ON | OFF", "Flags"={"OPC Wait"=FALSE, "Dont check status"=FALSE, "*WAI"=FALSE}, "Check Status Callback"=""}, {"Level"=2, "Descriptive Name"="NWA Alarm Sound State", "Class Only"=FALSE, "Data Type"=3, "Access"=2, "Identifier"="RSZVL_ATTR_NWA_ALARM_SOUND_STATE", "Range Table"="", "Command"="SYST:SOUN:ALAR:STAT", "Read Callback"="", "Write Callback"="", "Range Callback"="", "Check Callback"="", "Rngtable Callback"="", "Coerce Callback"="", "User Callback"="", "Supported Models"="", "Instrument Options"="", "Repeated Capabilities"="", "Restricted Repeated Capabilities"="", "Help"="This attribute switches alarm sounds on or off.\n\nAvailable Repeated Capabilities:\nNone\n\nRemote-control command(s):\nSYSTem:SOUNd:ALARm[:STATe] ON | OFF", "Flags"={"OPC Wait"=FALSE, "Dont check status"=FALSE, "*WAI"=FALSE}, "Check Status Callback"=""}, {"Level"=2, "Descriptive Name"="NWA Status Sound State", "Class Only"=FALSE, "Data Type"=3, "Access"=2, "Identifier"="RSZVL_ATTR_NWA_STATUS_SOUND_STATE", "Range Table"="", "Command"="SYST:SOUN:STAT:STAT", "Read Callback"="", "Write Callback"="", "Range Callback"="", "Check Callback"="", "Rngtable Callback"="", "Coerce Callback"="", "User Callback"="", "Supported Models"="", "Instrument Options"="", "Repeated Capabilities"="", "Restricted Repeated Capabilities"="", "Help"="This attribute switches status sounds on or off.\n\nAvailable Repeated Capabilities:\nNone\n\nRemote-control command(s):\nSYSTem:SOUNd:STATus[:STATe] ON | OFF", "Flags"={"OPC Wait"=FALSE, "Dont check status"=FALSE, "*WAI"=FALSE}, "Check Status Callback"=""}, {"Level"=2, "Descriptive Name"="NWA Unit Of Length", "Class Only"=FALSE, "Data Type"=0, "Access"=2, "Identifier"="RSZVL_ATTR_NWA_UNIT_OF_LENGTH", "Range Table"="rszvl_rngUnitLength", "Command"="UNIT:LENG", "Read Callback"="", "Write Callback"="", "Range Callback"="", "Check Callback"="", "Rngtable Callback"="", "Coerce Callback"="", "User Callback"="", "Supported Models"="", "Instrument Options"="", "Repeated Capabilities"="", "Restricted Repeated Capabilities"="", "Help"="This attribute defines the default unit of length. The command affects all SCPI commands defining a parameter with a physical unit that is related to a length, in particular: \n\n- Length offset parameters ([SENSe:]CORRection:EDELay...) \n- Parameters of the distance-to fault measurement (CALCulate<Chn>:TRANSform:DTFault...) \n- Derived units, e.g. the attenuation per unit of length defined via CALCulate<Ch>:TRANsform:DTFault:DEFine \n- Stimulus values for limit lines and ripple limit lines for the distance-to fault trace (e.g. CALCulate<Chn>:LIMit:DATA)\n\nMETer – metric units \nFOOT – foot (ft). 1 foot corresponds to 0.3048 m (1 m = 3.28084 ft)\n\nAvailable Repeated Capabilities:\nNone\n\nRemote-control command(s):\nUNIT:LENGth METer | FOOT", "Flags"={"OPC Wait"=FALSE, "Dont check status"=FALSE, "*WAI"=FALSE}, "Check Status Callback"=""}, {"Level"=1, "Descriptive Name"="K7 - FM Demodulator", "Class Only"=TRUE, "Data Type"=0, "Access"=0, "Identifier"="", "Range Table"="", "Command"="", "Read Callback"="", "Write Callback"="", "Range Callback"="", "Check Callback"="", "Rngtable Callback"="", "Coerce Callback"="", "User Callback"="", "Supported Models"="", "Instrument Options"="", "Repeated Capabilities"="", "Restricted Repeated Capabilities"="", "Help"="This class defines attributes of FM Measurement Demodulator\n\n(1) FM Demod Mode:\nThis attribute switches instrument to FM demodulator mode.\n\n(2) FM Demod Trigger Source:\nThis attribute sets the FM Demodulation Trigger Source.\n\n(3) Analog Demod Trigger AM Level Abs:\nThis attribute sets the level when RF power signals are used as trigger source.\n\n(4) Analog Demod Trigger AM Level Relative:\nThis attribute sets the level when AM–modulated signals are used as trigger source.\n\n(5) Analog Demod Trigger FM Level:\nThis attribute sets the level when FM–modulated signals are used as trigger source.\n\n(6) Analog Demod Trigger PM Level:\nThis attribute sets the level when PM–modulated signals are used as trigger source.\n\n(7) Settings (Class):\nAttributes that configures the common settings of FM Demodulator.\n\n(8) AF Frequency Settings (Class):\nAttributes that configures the AF Frequency settings.\n\n(9) RF Spectrum Settings (Class):\nAttributes that configures the RF Spectrum settings.\n\n(10) AF Filter Settings (Class):\nAttributes that configures the AF Filter settings.\n\n(11) Results (Class):\nAttributes that return the measurement results.", "Flags"={"OPC Wait"=FALSE, "Dont check status"=FALSE, "*WAI"=FALSE}, "Check Status Callback"=""}, {"Level"=2, "Descriptive Name"="FM Demod Mode", "Class Only"=FALSE, "Data Type"=4, "Access"=1, "Identifier"="RSZVL_ATTR_FMDEM_MODE", "Range Table"="", "Command"="INST ADEM", "Read Callback"="", "Write Callback"="", "Range Callback"="", "Check Callback"="", "Rngtable Callback"="", "Coerce Callback"="", "User Callback"="", "Supported Models"="", "Instrument Options"="", "Repeated Capabilities"="", "Restricted Repeated Capabilities"="", "Help"="This attribute switches instrument to FM demodulator mode.\n\nAvailable Repeated Capabilities:\nNone\n\nRemote-control command(s):\nINSTrument[:SELect] ADEMod", "Flags"={"OPC Wait"=FALSE, "Dont check status"=FALSE, "*WAI"=FALSE}, "Check Status Callback"=""}, {"Level"=2, "Descriptive Name"="FM Demod Trigger Source", "Class Only"=FALSE, "Data Type"=0, "Access"=2, "Identifier"="RSZVL_ATTR_FMDEM_TRIGGER_SOURCE", "Range Table"="rszvl_rngFmTriggerSource", "Command"="TRIG:SOUR", "Read Callback"="", "Write Callback"="", "Range Callback"="", "Check Callback"="", "Rngtable Callback"="", "Coerce Callback"="", "User Callback"="", "Supported Models"="", "Instrument Options"="", "Repeated Capabilities"="", "Restricted Repeated Capabilities"="", "Help"="This attribute sets the FM Demodulation Trigger Source.\n\nAvailable Repeated Capabilities:\nNone\n\nRemote-control command(s):\nTRIGger<1|2>[:SEQuence]:SOURce IMMediate | EXTernal | IFPower | AF | FM | AM | PM", "Flags"={"OPC Wait"=FALSE, "Dont check status"=FALSE, "*WAI"=FALSE}, "Check Status Callback"=""}, {"Level"=2, "Descriptive Name"="Analog Demod Trigger AM Level Abs", "Class Only"=FALSE, "Data Type"=1, "Access"=2, "Identifier"="RSZVL_ATTR_ADEM_TRIGGER_AM_LEVEL_ABS", "Range Table"="rszvl_rngAdemTrigAMLevelAbs", "Command"="TRIG:LEV:AM", "Read Callback"="", "Write Callback"="", "Range Callback"="", "Check Callback"="", "Rngtable Callback"="", "Coerce Callback"="", "User Callback"="", "Supported Models"="", "Instrument Options"="", "Repeated Capabilities"="", "Restricted Repeated Capabilities"="", "Help"="This attribute sets the level when RF power signals are used as trigger source.\n\nAvailable Repeated Capabilities:\nNone\n\nRemote-control command(s):\nTRIGger<1|2>[:SEQuence]:LEVel:AM[:ABSolute]", "Flags"={"OPC Wait"=FALSE, "Dont check status"=FALSE, "*WAI"=FALSE}, "Check Status Callback"=""}, {"Level"=2, "Descriptive Name"="Analog Demod Trigger AM Level Relative", "Class Only"=FALSE, "Data Type"=1, "Access"=2, "Identifier"="RSZVL_ATTR_ADEM_TRIGGER_AM_LEVEL_REL", "Range Table"="rszvl_rngAdemTrigAMLevelRel", "Command"="TRIG:LEV:AM:REL", "Read Callback"="", "Write 
